vi "Weather Station UI.vi"() -> ()   [LabVIEW 2012]
doc: "表示气象站项目的主VI。其中包含用于温度警告系统的用户界面。每间隔半秒读取温度；发生警告时记录数据。"
uses:
  Supporting Files/Weather Station States.ctl
  Supporting Files/Weather Data.ctl
panel:
  out "警告":string
  in  "下限":dbl=20.0
  in  "上限":dbl=30.0
  in  "停止按钮":bool
  out "温度历史":dbl(graph)
  # "温度范围(C)"
  # "冷冻"
  # "中暑"
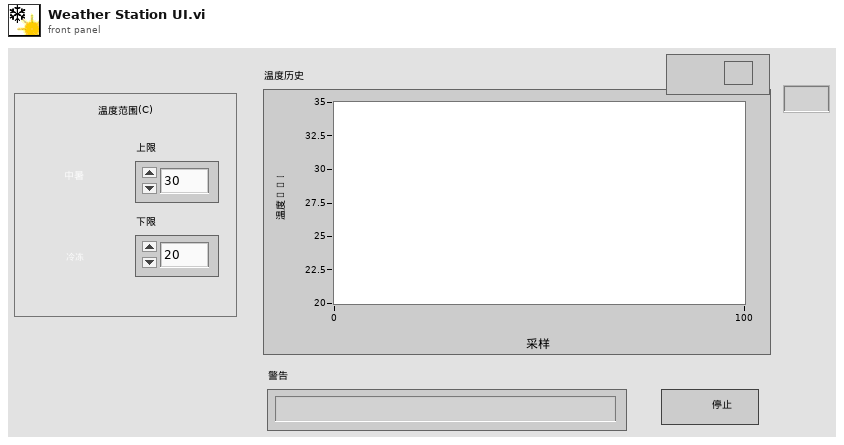
[diagram p1: front panel]
types:
  T1 = enum16{"open", "replace", "create", "open or create", "replace or create", "replace or create with confirmation"}
  T2 = typedef "Weather Data.ctl" = cluster{"当前温度":dbl, "最高温度":dbl, "最低温度":dbl, "温度警告？":bool, "温度警告文本":string}
  T3 = typedef "Weather Station States.ctl" = enum16{"采集", "范围检查", "分析", "数据记录", "时间检查"}
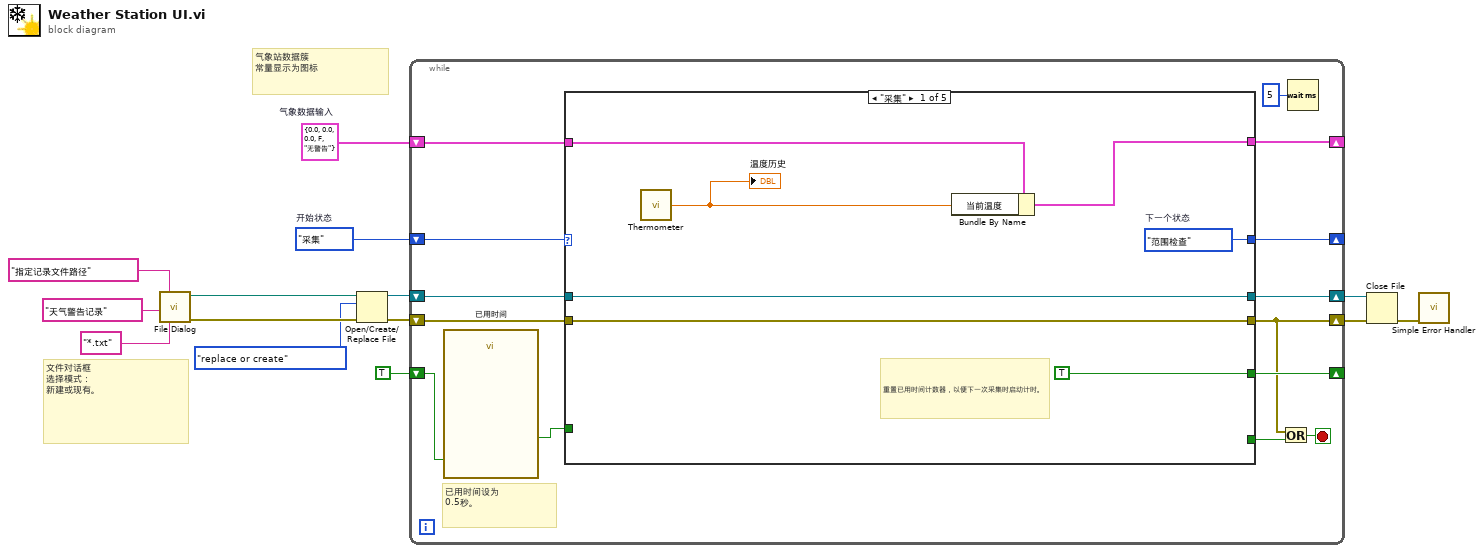
[diagram p0: block diagram]
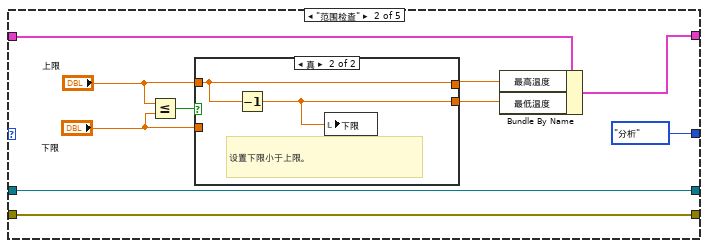
[diagram p2: hidden frame]
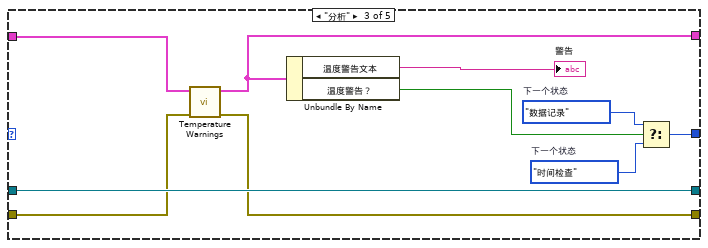
[diagram p4: hidden frame]
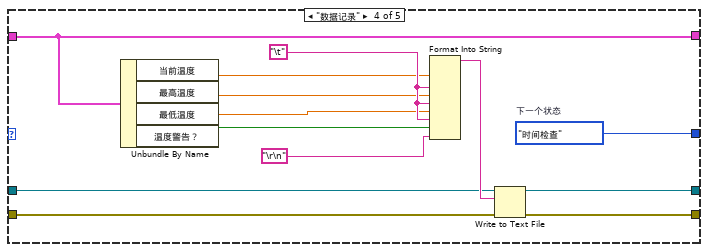
[diagram p5: hidden frame]
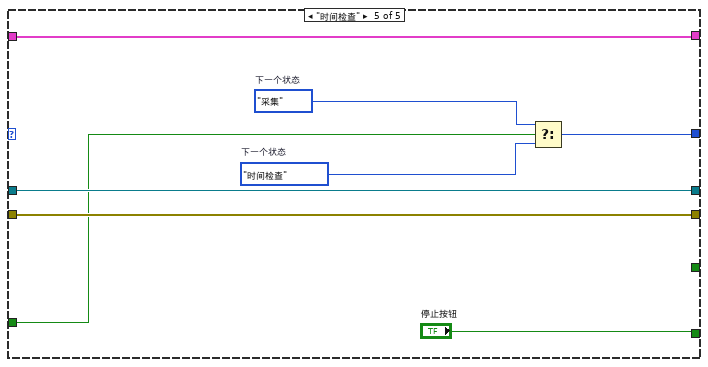
[diagram p6: hidden frame]
diagram:
  w7 = T2 {"当前温度"=0.0, "最高温度"=0.0, "最低温度"=0.0, "温度警告？"=FALSE, "温度警告文本"="无警告"}  # 气象数据输入
  w14 = Weather_Station_States."采集"  # 开始状态
  # "文件对话框\n选择模式：\n新建或现有。"
  # "气象站数据簇\n常量显示为图标"
  n1 = call "File Dialog"("prompt"="指定记录文件路径" ("提示"), "default name"="天气警告记录" ("默认名称"), "pattern (all files)"="*.txt" ("类型标签")) -> ("selected path"=w6:path, "error out"=w3:errorcluster)  [unwired: 9 in, 2 out]
  n2 = Open/Create/Replace File ("打开/创建/替换文件")(file path (use dialog)=w6, error in=w3, operation (0:open)=T1."replace or create" ("操作(0:open)")) -> (refnum out=w9:refnum<file>, error out=w8:errorcluster)  [unwired: 3 in, 1 out]
  n3 = while {
    shift-right: [w27] -> _
    shift-left: w14 -> [w28]
    shift-right: [w15] -> w13
    shift-left: w8 -> [w26]
    shift-right: [w16] -> _
    shift-left: w7 -> [w23]
    shift-right: [w24] -> w12
    shift-left: w9 -> [w22]
    shift-right: [w17] -> _
    shift-left: TRUE ("停止") -> [w19]
    stop <- w25 stop-if-true
    # "已用时间设为\n0.5秒。"
    n4 = call "已用时间"("Reset"=w19) -> ("Time has Elapsed"=w18:bool)  [unwired: 11 in, 7 out]
    n5 = case shown="\"采集\"" w28 {
      tunnel: [w35 Weather_Station_States."分析" ("下一个状态") w53 w72 w73] -> w27
      tunnel: [w30 w45 w57 w70 w79] -> w15
      tunnel: w26 -> [w30 w45 w58 w71 w79]
      tunnel: [w34 w44 w59 w69 w80] -> w24
      tunnel: [w31 w41 w52 w60 w78] -> w16
      tunnel: w23 -> [w32 w42 w50 w60 w78]
      tunnel: w22 -> [w34 w44 w59 w67 w80]
      tunnel: [_ _ _ _ "停止按钮"] -> w21
      tunnel: w18 -> [_ _ _ _ w74]
      tunnel: [TRUE ("停止") _ _ _ _] -> w17
      frame "采集" {
        w35 = Weather_Station_States."范围检查"  # 下一个状态
        # "重置已用时间计数器，以便下一次采集时启动计时。"
        n6 = call "Thermometer.vi"() -> ("温度"=w29:dbl)  [unwired: 1 in]
        "温度历史" <- w29
        n7 = Bundle By Name ("按名称捆绑")(cluster=w32, "当前温度"=w29) -> (w31:T2)
      }
      frame "范围检查" {
        n8 = Less Or Equal? ("小于等于？")(x="上限", y="下限") -> (x <= y?=w40:bool)
        n9 = case shown="真" w40 {
          tunnel: "上限" -> [w47 w49]
          tunnel: "下限" -> [w46 _]
          tunnel: [w47 w49] -> w37
          tunnel: [w46 w48] -> w36
          frame False {
          }
          frame True {
            # "设置下限小于上限。"
            n10 = Decrement ("减1")(x=w49) -> (x-1=w48:dbl)
            n11 = local write "下限"(w48) -> ()
          }
        }
        n12 = Bundle By Name ("按名称捆绑")(cluster=w42, "最高温度"=w37, "最低温度"=w36) -> (w41:T2)
      }
      frame "分析" {
        w55 = Weather_Station_States."数据记录"  # 下一个状态
        w54 = Weather_Station_States."时间检查"  # 下一个状态
        n13 = call "Temperature Warnings.vi"("错误输入"=w58, "气象数据输入"=w50) -> ("错误输出"=w57:cluster{"状态":bool, "代码":i32, "源":string}, "气象数据输出"=w52:T2)  [unwired: 8 in]
        n14 = Unbundle By Name ("按名称解除捆绑")(w52) -> ("温度警告文本"=→"警告":string, "温度警告？"=w56:bool)
        n15 = Select ("选择")(t=w55, s=w56, f=w54) -> (s? t:f=w53:T3)
      }
      frame "数据记录" {
        w72 = Weather_Station_States."时间检查"  # 下一个状态
        w66 = "\t" ("制表符常量")
        n16 = Unbundle By Name ("按名称解除捆绑")(w60) -> ("当前温度"=w65:dbl, "最高温度"=w64:dbl, "最低温度"=w63:dbl, "温度警告？"=w62:bool)
        n17 = Format Into String ("格式化写入字符串")(w65, w66, w64, w66, w63, w66, w62, "\r\n" ("行结束常量")) -> (resulting string=w68:string)  [unwired: 3 in, 1 out]
        n18 = Write to Text File ("写入文本文件")(file (use dialog)=w67, text=w68, error in=w71) -> (refnum out=w69:refnum<file>, error out=w70:errorcluster)  [unwired: 1 in, 1 out]
      }
      frame "时间检查" {
        w76 = Weather_Station_States."时间检查"  # 下一个状态
        w75 = Weather_Station_States."采集"  # 下一个状态
        n19 = Select ("选择")(t=w75, s=w74, f=w76) -> (s? t:f=w73:T3)
      }
    }
    n20 = Or ("或")(x=w15, y=w21) -> (x .or. y?=w25:bool)
    n21 = Wait (ms) ("等待(ms)")(milliseconds to wait=u32 5 ("y")) -> ()  [unwired: 1 out]
  }
  n22 = Close File ("关闭文件")(refnum=w12, error in=w13) -> (error out=w11:errorcluster)  [unwired: 1 out]
  n23 = call <vilib>:"Simple Error Handler.vi"("error in (no error)"=w11) -> ()  [unwired: 4 in, 5 out]
